vi "rad_Add FPGA Properties to INI.vi"(7 "section":string, 8 "error in (no error)":errorcluster, 10 "FPGA Properties":T2, 11 "refnum in":T1) -> (0 "error out":errorcluster, 3 "refnum out":T1)   [LabVIEW 2016]
uses:
  TypeDefs/rad_FPGA Properties.ctl
  TypeDefs/rad_FPGA Flash Properties.ctl
  <vilib>/Utility/config.llb/Config Data RefNum.ctl
  <vilib>/Utility/config.llb/Write Key (I32).vi
  <vilib>/Utility/config.llb/Write Key (String).vi
  <vilib>/Utility/config.llb/NI_LVConfig.lvlib
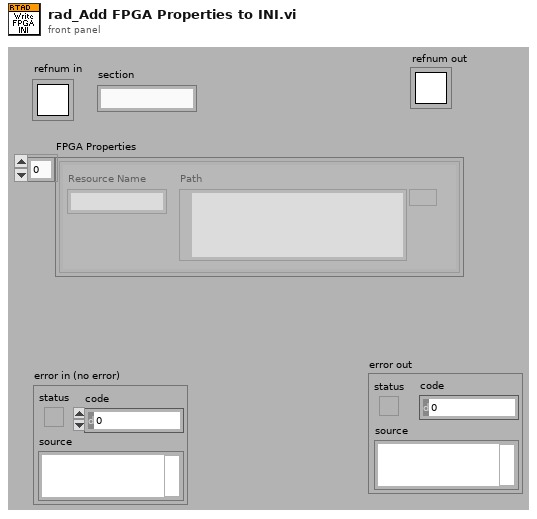
[diagram p1: front panel]
types:
  T1 = typedef "NI_LVConfig.lvlib/Config Data RefNum.ctl" = refnum<k1>
  T2 = typedef "rad_FPGA Properties.ctl" = T3[]
  T3 = typedef "rad_FPGA Flash Properties.ctl" = cluster{"Resource Name":string, "Path":path}
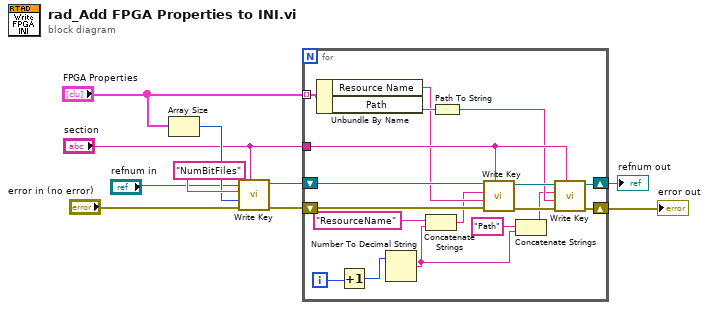
[diagram p0: block diagram]
diagram:
  n1 = Array Size(array="FPGA Properties") -> (size(s)=w6:i32)
  n2 = call-poly <vilib>:"Write Key.vi"("section"="section", "error in (no error)"="error in (no error)", "value"=w6, "key"="NumBitFiles", "refnum"="refnum in") -> ("error out"=w9:errorcluster, "refnum out"=w10:T1)  [unwired: 4 in, 1 out]
  n3 = for {
    tunnel: "FPGA Properties" -> [w28] mode=indexing
    tunnel: "section" -> [w24]
    shift-right: [w21] -> w1
    shift-left: w10 -> [w26]
    shift-right: [w18] -> w2
    shift-left: w9 -> [w20]
    i -> [w17]
    n4 = Unbundle By Name(w28) -> ("Resource Name"=w23:string, "Path"=w27:path)
    n5 = Increment(x=w17) -> (x+1=w16:i32)
    n6 = Number To Decimal String(number=w16) -> (decimal integer string=w12:string)  [unwired: 1 in]
    n7 = Concatenate Strings("ResourceName" ("key"), w12) -> (w14:string)
    n8 = Path To String(path=w27) -> (string=w22:string)
    n9 = call-poly <vilib>:"Write Key.vi"("section"=w24, "error in (no error)"=w20, "value"=w23, "key"=w14, "refnum"=w26) -> ("error out"=w19:errorcluster, "refnum out"=w25:T1)  [unwired: 4 in, 1 out]
    n10 = Concatenate Strings("Path" ("key"), w12) -> (w11:string)
    n11 = call-poly <vilib>:"Write Key.vi"("section"=w24, "error in (no error)"=w19, "value"=w22, "key"=w11, "refnum"=w25) -> ("error out"=w18:errorcluster, "refnum out"=w21:T1)  [unwired: 4 in, 1 out]
  }
  "error out" <- w2
  "refnum out" <- w1
